vi "pack.vi"(8 "error in (no error)":errorcluster, 11 "DDSFileReader in":refnum<class "DDSFileReader.lvclass">) -> (0 "error out":errorcluster, 3 "DDSFileReader out":refnum<class "DDSFileReader.lvclass">)   [LabVIEW 2011, in "Tools.lvlib" / "Filing.lvlib" / "DDSFileReader.lvclass"]
uses:
  DDSFileReader.lvclass
  DDSFileReader.lvclass/DDSFileReader.ctl
  FileReader.lvclass
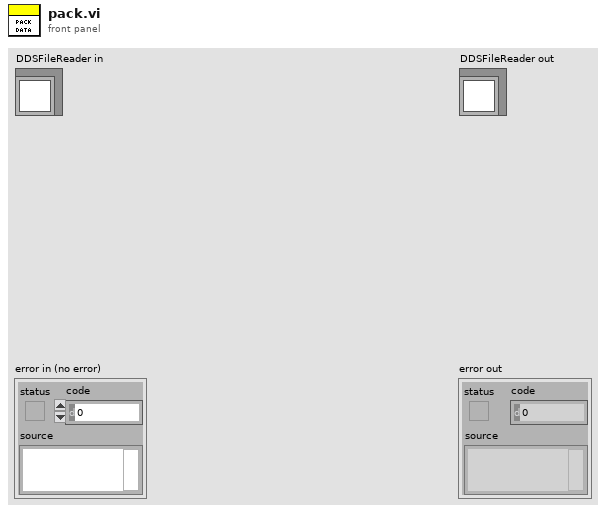
[diagram p1: front panel]
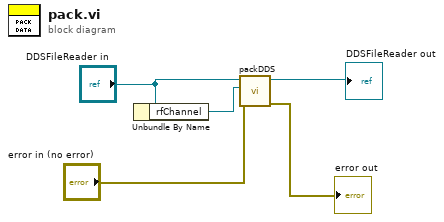
[diagram p0: block diagram]
diagram:
  n1 = Unbundle By Name("DDSFileReader in") -> ("rfChannel"=w4:refnum<class "DDSOutput.lvclass">)
  n2 = call "packDDS.vi"("error in (no error)"="error in (no error)", "rfChannel"=w4, "FileReader in"="DDSFileReader in") -> ("error out"=→"error out":errorcluster, "FileReader out"=→"DDSFileReader out":refnum<class "DDSFileReader.lvclass">)  [unwired: 7 in]
